vi "GetChannelList.vi"(8 "error in (no error)":errorcluster, 10 "asset code":string, 11 "ByteGSAPIBase in":refnum<class "ByteQXAPIBase.lvclass">) -> (0 "error out":errorcluster, 2 "channels":string[](array[string]), 3 "ByteGSAPIBase out":refnum<class "ByteQXAPIBase.lvclass">)   [LabVIEW 2019, in "ByteQXWebAPI.lvlib" / "ByteQXAPIBase.lvclass"]
uses:
  ByteQXAPIBase.lvclass
  GetChannels_ResData.ctl
  Private/module.ctl
  ByteQXAPIBase.lvclass/ByteQXAPIBase.ctl
  <vilib>/Bytelabs/ByteREST/ByteRESTClass/ByteRESTBase/RESTBase.lvclass
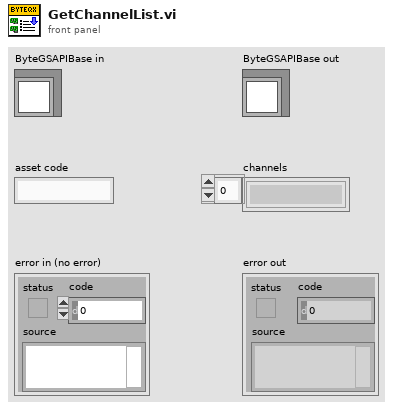
[diagram p1: front panel]
types:
  T1 = typedef "ByteQXWebAPI.lvlib/ByteQXAPIBase.lvclass/module.ctl" = enum16{"gs", "tms", "data"}
  T2 = typedef "ByteQXWebAPI.lvlib/ByteQXAPIBase.lvclass/GetChannels_ResData.ctl" = cluster{"fields":string[]}
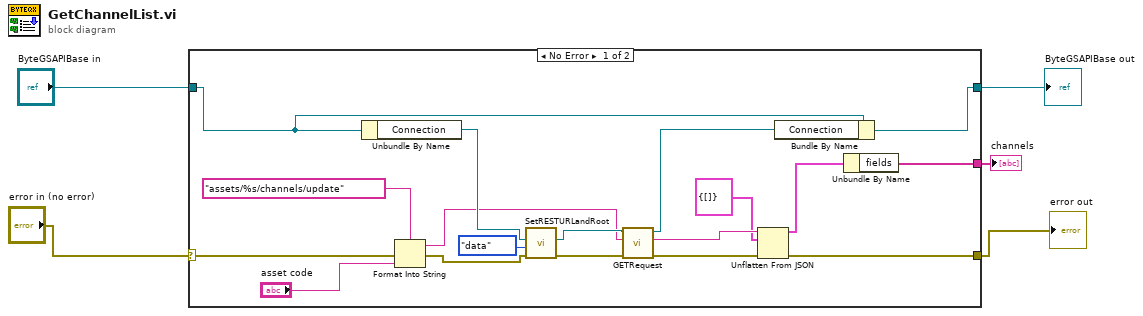
[diagram p0: block diagram]
diagram:
  n1 = case shown="No Error" "error in (no error)" {
    selector: "error in (no error)" -> [w10 w25]
    tunnel: [w18 w25] -> w3
    tunnel: [w22 w24] -> w2
    tunnel: "ByteGSAPIBase in" -> [w23 w24]
    tunnel: [w15 _] -> w1
    frame No Error {
      n2 = Unbundle By Name(w23) -> ("Connection"=w13:refnum<class "RESTBase.lvclass">)
      n3 = Format Into String(format string="assets/%s/channels/update" ("Request"), error in=w10, "asset code") -> (resulting string=w6:string, error out=w9:errorcluster)  [unwired: 1 in]
      n4 = call "SetRESTURLandRoot.vi"("error in (no error)"=w9, "module"=module."data", "ByteREST in"=w13) -> ("error out"=w11:errorcluster, "ByteREST out"=w12:refnum<class "RESTBase.lvclass">)  [unwired: 7 in]
      n5 = call-dynamic "GETRequest.vi"("error in (no error)"=w11, "Request"=w6, "ByteRESTBase in"=w12) -> ("error out"=w20:errorcluster, "Body"=w19:string, "ByteRESTBase out"=w21:refnum<class "RESTBase.lvclass">)  [unwired: 5 in, 1 out]
      n6 = Unflatten From JSON(JSON string=w19, type and defaults=T2 {"fields"=[]}, error in (no error)=w20) -> (value=w16:T2, error out=w18:errorcluster)  [unwired: 4 in]
      n7 = Bundle By Name(cluster=w23, "Connection"=w21) -> (w22:refnum<class "ByteQXAPIBase.lvclass">)
      n8 = Unbundle By Name(w16) -> ("fields"=w15:string[])
    }
    frame Error {
    }
  }
  "error out" <- w3
  "ByteGSAPIBase out" <- w2
  "channels" <- w1
